vi "monitor.vi"(3 "connection ID in":refnum<k5>, 4 "Received text 4":string, 5 "Received text 2":string) -> ()   [LabVIEW 2016]
uses:
  GrobaLimitVoltage.vi
panel:
  in  "stop":bool
  in  "Received text":string
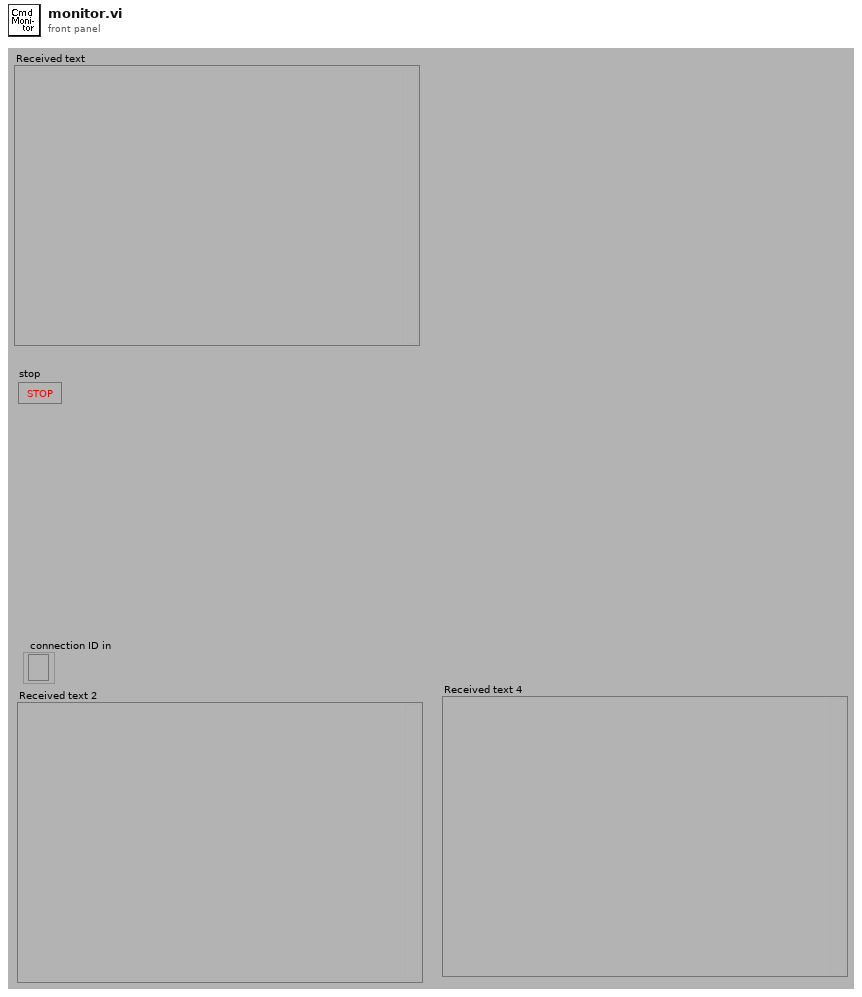
[diagram p1: front panel]
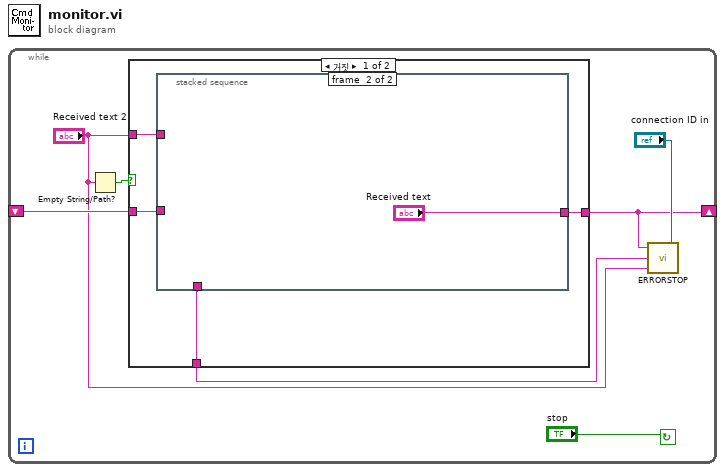
[diagram p0: block diagram]
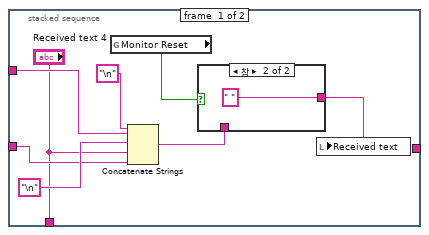
[diagram p2: hidden frame]
diagram:
  n1 = while {
    shift-right: [w1] -> _
    shift-left: _ -> [w7]
    stop <- "stop" continue-if-true
    n2 = Empty String/Path?(string/path="Received text 2") -> (empty?=w5:bool)
    n3 = case shown="거짓" w5 {
      tunnel: [w11 _] -> w1
      tunnel: w7 -> [w10 _]
      tunnel: "Received text 2" -> [w9 _]
      tunnel: [w8 _] -> w4
      frame False {
        n4 = stacked-sequence {
          tunnel: [_ "Received text"] -> w11
          tunnel: w10 -> [w16 _]
          tunnel: w9 -> [w18 _]
          tunnel: ["Received text 4" _] -> w8
          frame #0 {
            n5 = global read "GrobaLimitVoltage.vi" "Monitor Reset"() -> (w14:bool)
            n6 = Concatenate Strings("\n", w18, "\n", "Received text 4", w16) -> (w12:string)
            n7 = case shown="참" w14 {
              tunnel: [w20 " "] -> w13
              tunnel: w12 -> [w20 _]
              frame False {
              }
              frame True {
              }
            }
            n8 = local write "Received text"(w13) -> ()
          }
          frame #1 {
          }
        }
      }
      frame True {
      }
    }
    n9 = call "ERRORSTOP.vi"("connection ID in"="connection ID in", "Input Command"="Received text 2", "Received Command"=w4, "Total Command In/Output"=w1) -> ()  [unwired: 1 in]
  }
